vi "FileOutput-Start.vi"(3 "error in (no error)":errorcluster, 4 "OutputRequest\nuser event refnum":T1, 5 "Configuration":T2) -> (0 "error out":errorcluster)   [LabVIEW 2015]
doc: "Starts the FileOutput daemon running.\n\nIf an empty path or <Not a path> was specified in\nConfiguration.Logfile path\nthen this will deliver a message and exit."
uses:
  FileOutput-Configuration.ctl
  Typedefs/OutputRequest refnum.ctl
  Typedefs/OutputRequest.ctl
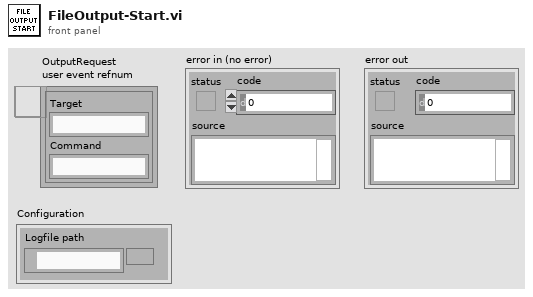
[diagram p1: front panel]
types:
  T1 = typedef "OutputRequest refnum.ctl" = refnum<user-event>
  T2 = typedef "FileOutput-Configuration.ctl" = cluster{"Logfile path":path}
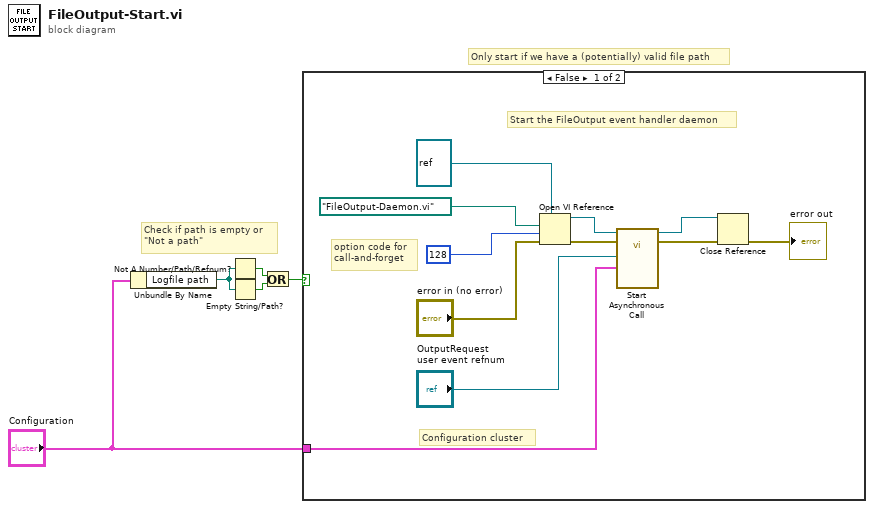
[diagram p0: block diagram]
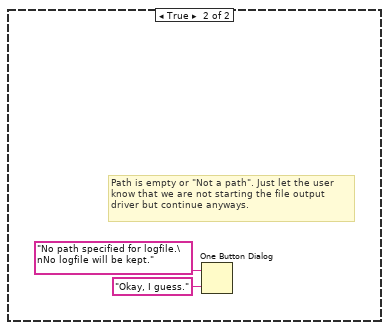
[diagram p2: hidden frame]
diagram:
  # "Only start if we have a (potentially) valid file path"
  # "Check if path is empty or\n\"Not a path\""
  n1 = Unbundle By Name("Configuration") -> ("Logfile path"=w1:path)
  n2 = Not A Number/Path/Refnum?(number/path/refnum=w1) -> (NaN/Path/Refnum?=w3:bool)
  n3 = Empty String/Path?(string/path=w1) -> (empty?=w4:bool)
  n4 = Or(x=w3, y=w4) -> (x .or. y?=w2:bool)
  n5 = case shown="False" w2 {
    tunnel: "Configuration" -> [w6 _]
    frame False {
      # "Configuration cluster"
      # "option code for\ncall-and-forget"
      # "Start the FileOutput event handler daemon"
      n6 = Open VI Reference(type specifier VI Refnum (for type only)=refnum<vi> refnum, vi path=path "FileOutput-Daemon.vi", options=128, error in (no error)="error in (no error)") -> (vi reference=w15:refnum<vi>, error out=w16:errorcluster)  [unwired: 2 in]
      n7 = call-by-ref "Start Asynchronous Call"(reference=w15, error in=w16, "Configuration"=w6, "OutputRequest\nuser event refnum"="OutputRequest\nuser event refnum") -> (reference out=w11:refnum<vi>, error out=w12:errorcluster)  [unwired: 3 in]
      n8 = Close Reference(reference=w11, error in (no error)=w12) -> (error out=→"error out":errorcluster)
    }
    frame True {
      # "Path is empty or \"Not a path\". Just let the user\nknow that we are not starting the file output\ndriver but continue anyways."
      n9 = One Button Dialog(message="No path specified for logfile.\nNo logfile will be kept.", button name ("OK")="Okay, I guess.") -> ()  [unwired: 1 out]
    }
  }
